vi "TrajectoryState_ApproxEquals.vi"(6 "Tolerance":T1={"TimeSeconds"=0.005, "Velocity"=0.005, "Acceleration"=0.2, "POSE"={"TRANSLATION"={"X"=0.002, "Y"=0.002}, "ROTATION"={"VALUE"=0.002, "COS"=0.002, "SIN"=0.002}}, "Curvature"=0.3} {"POSE"."ROTATION"."SIN" format="%13.4f"; "POSE"."ROTATION"."COS" format="%13.4f"; "POSE"."ROTATION"."VALUE" format="%13.4f"; "POSE"."TRANSLATION"."Y" format="%14.3f"; "POSE"."TRANSLATION"."X" format="%14.3f"}, 9 "Other TRAJ_STATE":T1={"TimeSeconds"=0.0, "Velocity"=0.0, "Acceleration"=0.0, "POSE"={"TRANSLATION"={"X"=0.0, "Y"=0.0}, "ROTATION"={"VALUE"=0.0, "COS"=1.0, "SIN"=0.0}}, "Curvature"=0.0} {"POSE"."ROTATION"."SIN" format="%13.4f"; "POSE"."ROTATION"."COS" format="%13.4f"; "POSE"."ROTATION"."VALUE" format="%13.4f"; "POSE"."TRANSLATION"."Y" format="%14.3f"; "POSE"."TRANSLATION"."X" format="%14.3f"}, 11 "TRAJ_STATE":T1={"TimeSeconds"=0.0, "Velocity"=0.0, "Acceleration"=0.0, "POSE"={"TRANSLATION"={"X"=0.0, "Y"=0.0}, "ROTATION"={"VALUE"=0.0, "COS"=1.0, "SIN"=0.0}}, "Curvature"=0.0} {"POSE"."ROTATION"."SIN" format="%13.4f"; "POSE"."ROTATION"."COS" format="%13.4f"; "POSE"."ROTATION"."VALUE" format="%13.4f"; "POSE"."TRANSLATION"."Y" format="%14.3f"; "POSE"."TRANSLATION"."X" format="%14.3f"}) -> (3 "Equals":bool)   [LabVIEW 2019]
doc: "Determines if two Trajectory States are equal\n \nParameters:\n - TrajState - TrajectoryState data structure\n - Other TrajState - Other TrajectoryState data structure\n \nReturns:\n - Equals - boolean indicating if the states are equal."
uses:
  <vilib>/Rock Robotics/WPI/ThirdParty/JAS_Junk/TrajLib/TRAJ_STATE.ctl
  <vilib>/Rock Robotics/WPI/ThirdParty/JAS_Junk/TrajLib/POSE2D.ctl
  <vilib>/Rock Robotics/WPI/ThirdParty/JAS_Junk/TrajLib/TRANSLATION2D.ctl
  <vilib>/Rock Robotics/WPI/ThirdParty/JAS_Junk/TrajLib/ROTATION2D.ctl
  <vilib>/Rock Robotics/WPI/ThirdParty/JAS_Junk/TrajLib/Trajectory_Library.lvlib
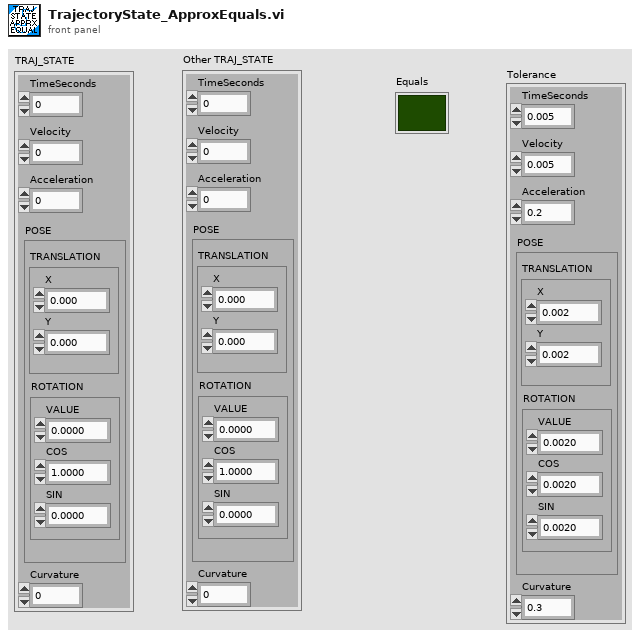
[diagram p1: front panel]
types:
  T1 = typedef "Trajectory_Library.lvlib/TRAJ_STATE.ctl" = cluster{"TimeSeconds":dbl, "Velocity":dbl, "Acceleration":dbl, "POSE":T2, "Curvature":dbl}
  T2 = typedef "Trajectory_Library.lvlib/POSE2D.ctl" = cluster{"TRANSLATION":T3, "ROTATION":T4}
  T3 = typedef "Trajectory_Library.lvlib/TRANSLATION2D.ctl" = cluster{"X":dbl, "Y":dbl}
  T4 = typedef "Trajectory_Library.lvlib/ROTATION2D.ctl" = cluster{"VALUE":dbl, "COS":dbl, "SIN":dbl}
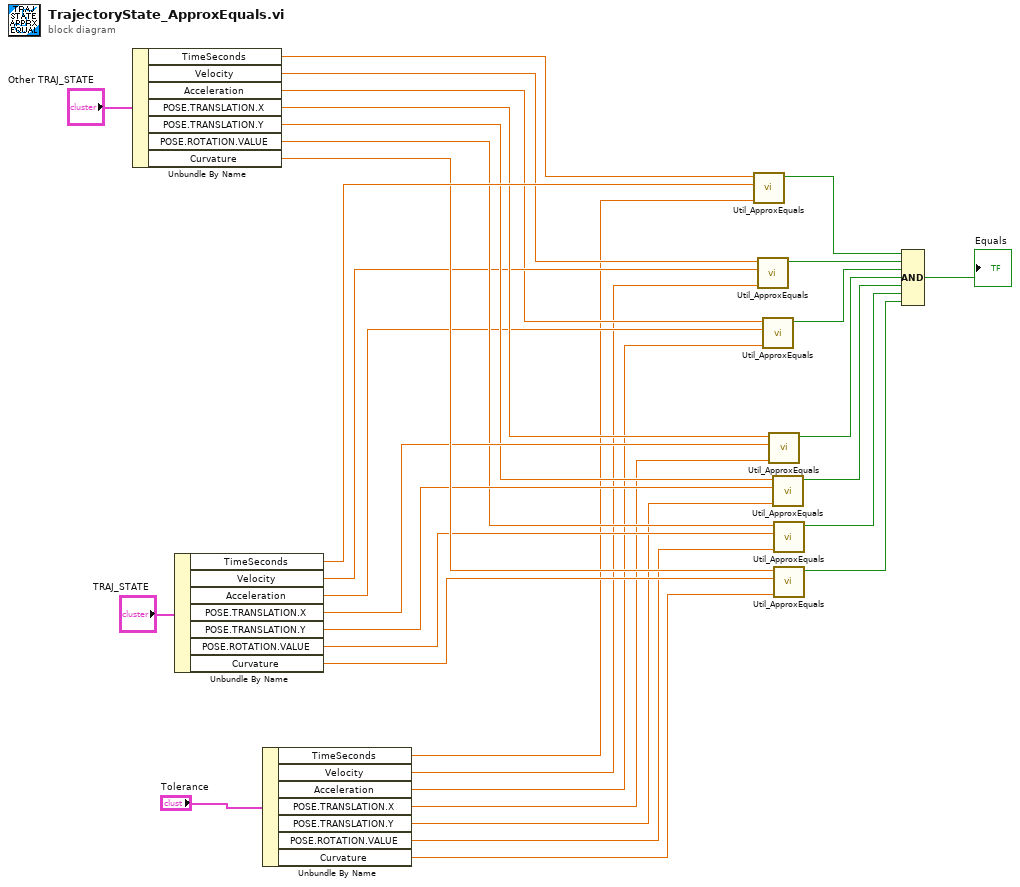
[diagram p0: block diagram]
diagram:
  n1 = Unbundle By Name("Other TRAJ_STATE") -> ("TimeSeconds"=w28:dbl, "Velocity"=w14:dbl, "Acceleration"=w11:dbl, "POSE.TRANSLATION.X"=w17:dbl, "POSE.TRANSLATION.Y"=w16:dbl, "POSE.ROTATION.VALUE"=w15:dbl, "Curvature"=w26:dbl)
  n2 = Unbundle By Name("TRAJ_STATE") -> ("TimeSeconds"=w27:dbl, "Velocity"=w13:dbl, "Acceleration"=w10:dbl, "POSE.TRANSLATION.X"=w21:dbl, "POSE.TRANSLATION.Y"=w22:dbl, "POSE.ROTATION.VALUE"=w23:dbl, "Curvature"=w25:dbl)
  n3 = Unbundle By Name("Tolerance") -> ("TimeSeconds"=w7:dbl, "Velocity"=w6:dbl, "Acceleration"=w5:dbl, "POSE.TRANSLATION.X"=w4:dbl, "POSE.TRANSLATION.Y"=w3:dbl, "POSE.ROTATION.VALUE"=w2:dbl, "Curvature"=w1:dbl)
  n4 = call <vilib>:"Util_ApproxEquals.vi"("Tolerance"=w7, "Value 2"=w27, "Value 1"=w28) -> ("ApproxEquals"=w30:bool)  [unwired: 8 in]
  n5 = call <vilib>:"Util_ApproxEquals.vi"("Tolerance"=w6, "Value 2"=w13, "Value 1"=w14) -> ("ApproxEquals"=w12:bool)  [unwired: 8 in]
  n6 = call <vilib>:"Util_ApproxEquals.vi"("Tolerance"=w5, "Value 2"=w10, "Value 1"=w11) -> ("ApproxEquals"=w9:bool)  [unwired: 8 in]
  n7 = call <vilib>:"Util_ApproxEquals.vi"("Tolerance"=w4, "Value 2"=w21, "Value 1"=w17) -> ("ApproxEquals"=w18:bool)  [unwired: 8 in]
  n8 = call <vilib>:"Util_ApproxEquals.vi"("Tolerance"=w3, "Value 2"=w22, "Value 1"=w16) -> ("ApproxEquals"=w19:bool)  [unwired: 8 in]
  n9 = call <vilib>:"Util_ApproxEquals.vi"("Tolerance"=w2, "Value 2"=w23, "Value 1"=w15) -> ("ApproxEquals"=w20:bool)  [unwired: 8 in]
  n10 = call <vilib>:"Util_ApproxEquals.vi"("Tolerance"=w1, "Value 2"=w25, "Value 1"=w26) -> ("ApproxEquals"=w24:bool)  [unwired: 8 in]
  n11 = Compound Arithmetic op=AND(w30, w12, w9, w18, w19, w20, w24) -> (→"Equals":bool)
